vi "TDMS_Convert_Version.vi"() -> ()   [LabVIEW 2019]
panel:
  in  "File Path":path
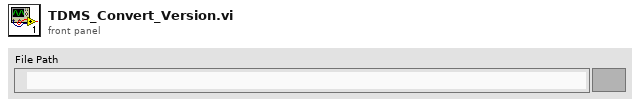
[diagram p1: front panel]
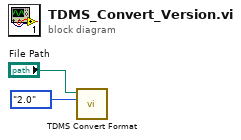
[diagram p0: block diagram]
diagram:
  n1 = call <vilib>:"TDMS Convert Format.vi"("target version"=enum16{"1.0", "2.0"}."2.0", "file path"="File Path") -> ()  [unwired: 4 in, 2 out]
